vi "KinectCode.vi"() -> ()   [LabVIEW 2013]
uses:
  <vilib>/addons/Kinect/Skeleton Vertex Index.ctl
  <vilib>/addons/Kinect/SkeletonVertexTrackState.ctl
panel:
  out "NumPlayers":i8
  out "Hot?":bool
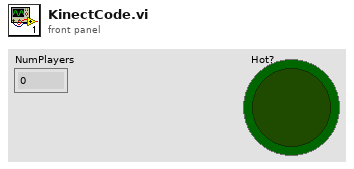
[diagram p1: front panel]
types:
  T1 = typedef "SkeletonVertexTrackState.ctl" = enum32{"NotTracked", "Inferred", "Tracked"}
  T2 = typedef "Skeleton Vertex Index.ctl" = i32
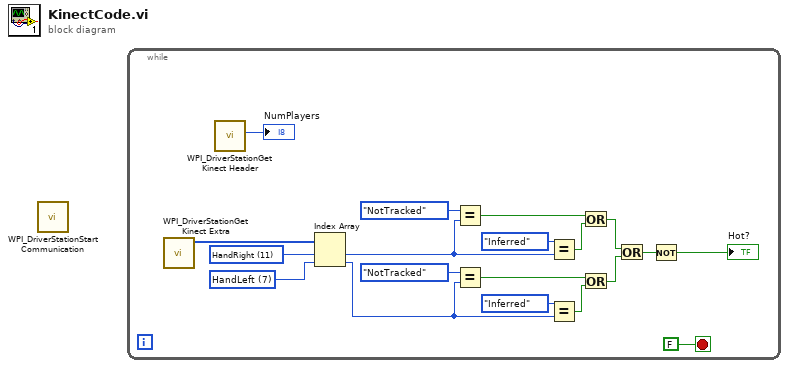
[diagram p0: block diagram]
diagram:
  n1 = call <vilib>:"WPI_DriverStationStart Communication.vi"() -> ()  [unwired: 12 in]
  n2 = while {
    stop <- FALSE stop-if-true
    w17 = T2 7 items=["HipCenter", "Spine", "ShoulderCenter", "Head", "ShoulderLeft", "ElbowLeft", "WristLeft", "HandLeft", "ShoulderRight", "ElbowRight", "WristRight", "HandRight", "HipLeft", "KneeLeft", "AnkleLeft", "FootLeft", "HipRight", "KneeRight", "AnkleRight", "FootRight"] ("Skeleton Joints")
    w18 = T2 11 items=["HipCenter", "Spine", "ShoulderCenter", "Head", "ShoulderLeft", "ElbowLeft", "WristLeft", "HandLeft", "ShoulderRight", "ElbowRight", "WristRight", "HandRight", "HipLeft", "KneeLeft", "AnkleLeft", "FootLeft", "HipRight", "KneeRight", "AnkleRight", "FootRight"] ("Skeleton Joints")
    n3 = call <vilib>:"WPI_DriverStationGet Kinect Extra.vi"() -> ("Skeleton Tracking State"=w19:T1[])  [unwired: 7 in, 4 out]
    n4 = call <vilib>:"WPI_DriverStationGet Kinect Header.vi"() -> ("NumPlayers"=→"NumPlayers":i8)  [unwired: 6 in, 5 out]
    n5 = Index Array(array=w19, index #1=w18, index #2=w17) -> (element #1=w15:T1, element #2=w7:T1)
    n6 = Equal?(x=SkeletonVertexTrackState."NotTracked" ("element"), y=w15) -> (x = y?=w12:bool)
    n7 = Equal?(x=SkeletonVertexTrackState."NotTracked" ("element"), y=w7) -> (x = y?=w8:bool)
    n8 = Equal?(x=SkeletonVertexTrackState."Inferred" ("element"), y=w15) -> (x = y?=w13:bool)
    n9 = Equal?(x=SkeletonVertexTrackState."Inferred" ("element"), y=w7) -> (x = y?=w9:bool)
    n10 = Or(x=w12, y=w13) -> (x .or. y?=w4:bool)
    n11 = Or(x=w8, y=w9) -> (x .or. y?=w3:bool)
    n12 = Or(x=w4, y=w3) -> (x .or. y?=w2:bool)
    n13 = Not(x=w2) -> (.not. x?=→"Hot?":bool)
  }
